vi "Get Time from String.vi"(11 "DataIn":string) -> (3 "time stamp":timestamp)   [LabVIEW 2013, in "Airmar Data.lvclass"]
uses:
  Airmar Data.lvclass
  <vilib>/Utility/miscctls.llb/LVDateTimeRec.ctl
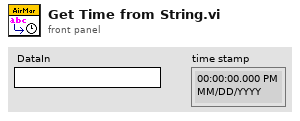
[diagram p1: front panel]
types:
  T1 = typedef "LVDateTimeRec.ctl" = cluster{"fractional second":dbl, "second":i32, "minute":i32, "hour":i32, "day of month":i32, "month":i32, "year":i32, "day of week":i32, "day of year":i32, "DST":i32}
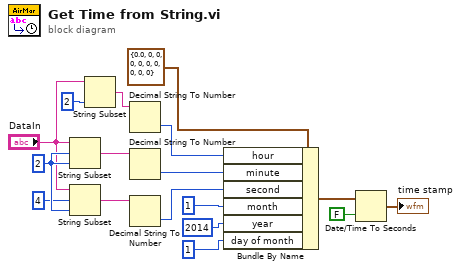
[diagram p0: block diagram]
diagram:
  w12 = 2 ("offset")
  n1 = String Subset(string="DataIn", offset (0)=w12, length (rest)=w12) -> (substring=w9:string)
  n2 = String Subset(string="DataIn", offset (0)=4 ("offset"), length (rest)=w12) -> (substring=w13:string)
  n3 = String Subset(string="DataIn", length (rest)=2 ("length (rest)")) -> (substring=w3:string)  [unwired: 1 in]
  n4 = Decimal String To Number(string=w3) -> (number=w4:i32)  [unwired: 2 in, 1 out]
  n5 = Decimal String To Number(string=w9) -> (number=w5:i32)  [unwired: 2 in, 1 out]
  n6 = Decimal String To Number(string=w13) -> (number=w14:i32)  [unwired: 2 in, 1 out]
  n7 = Bundle By Name(cluster=T1 {"fractional second"=0.0, "second"=0, "minute"=0, "hour"=0, "day of month"=0, "month"=0, "year"=0, "day of week"=0, "day of year"=0, "DST"=0} ("date time rec"), "hour"=w4, "minute"=w5, "second"=w14, "month"=1, "year"=2014, "day of month"=1) -> (w6:T1)
  n8 = Date/Time To Seconds(1:FALSE ("is UTC (F)"), 2:w6) -> (0:→"time stamp":timestamp)
